vi "Read User Name.vi"(8 "error in (no error)":errorcluster, 11 "SysCfg Device in":refnum<class "SysCfg Device.lvclass">) -> (0 "error out":errorcluster, 2 "User Name":string, 3 "SysCfg Device out":refnum<class "SysCfg Device.lvclass">)   [LabVIEW 2015, in "SMI.lvlib" / "SysCfg Device.lvclass"]
uses:
  SysCfg Device.lvclass
  SysCfg Device.lvclass/SysCfg Device.ctl
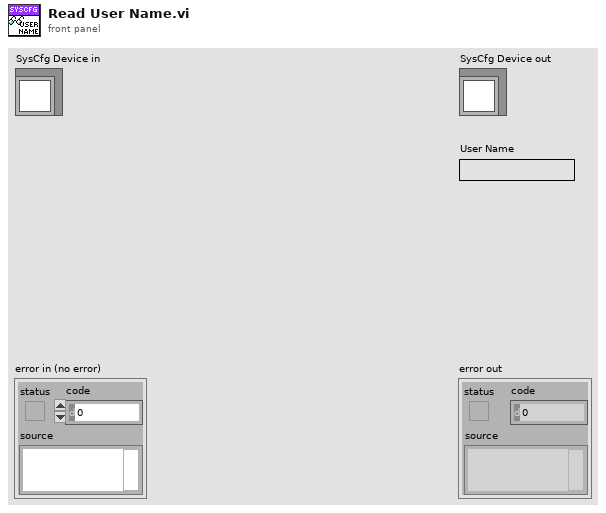
[diagram p1: front panel]
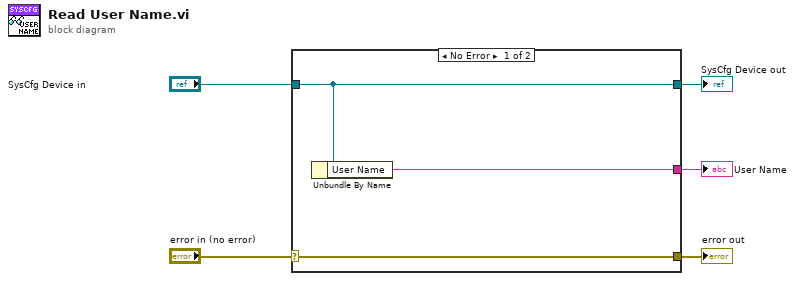
[diagram p0: block diagram]
diagram:
  n1 = case shown="No Error" "error in (no error)" {
    selector: "error in (no error)" -> [w8 w9]
    tunnel: [w8 w9] -> w4
    tunnel: [w7 w10] -> w2
    tunnel: "SysCfg Device in" -> [w7 w10]
    tunnel: [w6 _] -> w1
    frame No Error {
      n2 = Unbundle By Name(w7) -> ("User Name"=w6:string)
    }
    frame Error {
    }
  }
  "error out" <- w4
  "SysCfg Device out" <- w2
  "User Name" <- w1
